vi "Stop n Log.vi"(7 "Object in":refnum<class>, 8 "error in (no error)":errorcluster, 11 "Speedometer in":refnum<class "Speedometer.lvclass">) -> (0 "error out":errorcluster)   [LabVIEW 2026, in "TALOS.lvlib" / "Classes.lvlib" / "Speedometer.lvclass"]
uses:
  Speedometer.lvclass
  Speedometer.lvclass/Speedometer.ctl
  TALOS.lvlib
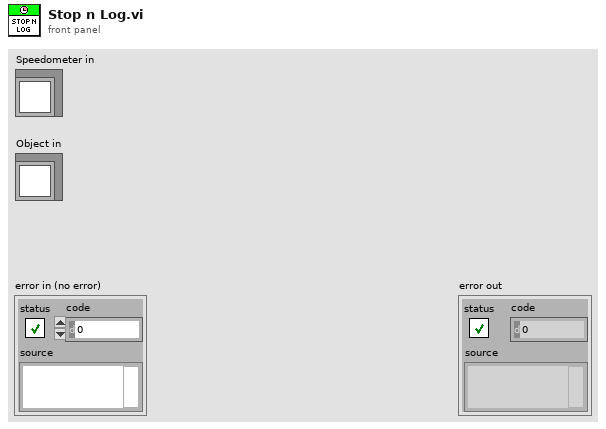
[diagram p1: front panel]
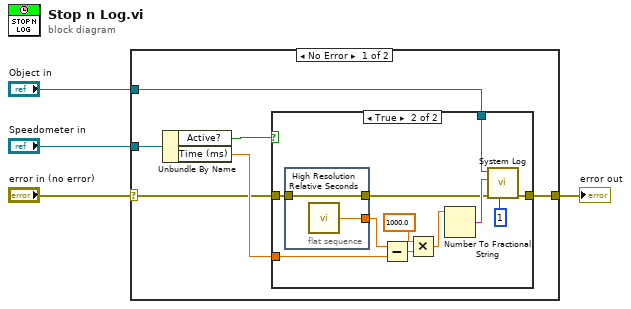
[diagram p0: block diagram]
diagram:
  n1 = case shown="No Error" "error in (no error)" {
    selector: "error in (no error)" -> [w7 w25]
    tunnel: [w6 w25] -> w3
    tunnel: "Speedometer in" -> [w10 _]
    tunnel: "Object in" -> [w5 _]
    frame No Error {
      n2 = Unbundle By Name(w10) -> ("Active?"=w9:bool, "Time (ms)"=w8:dbl)
      n3 = case shown="True" w9 {
        tunnel: w8 -> [_ w21]
        tunnel: [w11 w20] -> w6
        tunnel: w7 -> [w11 w15]
        tunnel: w5 -> [_ w12]
        frame False {
        }
        frame True {
          n4 = flat-sequence {
            tunnel: [w24] -> w22
            tunnel: w15 -> [w23]
            tunnel: [w23] -> w14
            frame #0 {
              n5 = call <vilib>:"High Resolution Relative Seconds.vi"() -> ("relative seconds"=w24:dbl)
            }
          }
          n6 = Subtract(x=w22, y=w21) -> (x-y=w19:dbl)
          n7 = Multiply(x=1000.0, y=w19) -> (x*y=w17:dbl)
          n8 = Number To Fractional String(number=w17) -> (F-format string=w16:string)  [unwired: 3 in]
          n9 = call "System Log.vi"("VIs Hierarchy"=1, "error in (no error)"=w14, "Text to log"=w16, "Object in"=w12) -> ("error out"=w20:errorcluster)  [unwired: 7 in]
        }
      }
    }
    frame Error {
    }
  }
  "error out" <- w3
